vi "PPR_Teleop_System_Execute.vi"(11 "Teleop Elapsed Seconds":dbl) -> ()   [LabVIEW 2019]
uses:
  <vilib>/Rock Robotics/WPI/Joystick/XBox Buttons Indexer.ctl
  <vilib>/Rock Robotics/WPI/Joystick/XBox Axes Indexer.ctl
  <vilib>/Rock Robotics/WPI/ThirdParty/JAS_Junk/TrajLib/Rotation2d_CreateAngle.vi
  <vilib>/Rock Robotics/WPI/ThirdParty/JAS_Junk/TrajLib/Translation2d_Create.vi
  <vilib>/Rock Robotics/WPI/ThirdParty/JAS_Junk/TrajLib/VI/Util_GetTime_U32.vi
  <vilib>/Rock Robotics/WPI/ThirdParty/JAS_Junk/TrajLib/VI/BoolCmd_Send_Internal.vi
  <vilib>/Rock Robotics/WPI/ThirdParty/JAS_Junk/TrajLib/VI/numCmd_ObtainQueue_TwoDbl.vi
  <vilib>/Rock Robotics/WPI/ThirdParty/JAS_Junk/TrajLib/VI/BoolCmd_ObtainQueue.vi
  <vilib>/Rock Robotics/WPI/ThirdParty/JAS_Junk/TrajLib/VI/Util_GetTime_U64.vi
  Diff_Drive_System/PPR_DRIVE_GLOBALS.vi
  <vilib>/Rock Robotics/WPI/Utilities/WPI_GetSetVariantRefNum.vi
  <vilib>/Rock Robotics/Network Tables/NT Write Integer Array.vi
  Trajectory Following/PPR_TRAJECTORY_GLOBALS.vi
  <vilib>/Rock Robotics/Network Tables/NT Write Numeric Array.vi
  <vilib>/Rock Robotics/WPI/Joystick/WPI_JoystickArcadeMapping.vi
  <vilib>/Rock Robotics/Network Tables/NT Write Boolean Array.vi
  <vilib>/Rock Robotics/WPI/ThirdParty/JAS_Junk/TrajLib/Trajectory_Library.lvlib
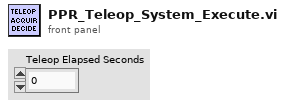
[diagram p1: front panel]
types:
  T1 = typedef "XBox Buttons Indexer.ctl" = enum16{"A", "B", "X", "Y", "Left Bumper", "Right Bumper", "Back", "Start", "Left Joystick", "Right Joystick"}
  T2 = typedef "XBox Axes Indexer.ctl" = enum16{"Left X", "Left Y", "Left Trigger", "Right Trigger", "Right X", "Right Y"}
  T3 = typedef "WPI_JoystickDevRef.ctl" = cluster{"Device":T4}
  T4 = typedef "WPI_JoystickDeviceEnum.ctl" = enum16{"USB 0", "USB 1", "USB 2", "USB 3", "USB 4", "USB 5"}
  T5 = typedef "Trajectory_Library.lvlib/CHASSIS_SPEEDS.ctl" = cluster{"vX":dbl, "vY":dbl, "vOmega":dbl}
  T6 = typedef "Trajectory_Library.lvlib/POSE2D.ctl" = cluster{"TRANSLATION":T7, "ROTATION":T8}
  T7 = typedef "Trajectory_Library.lvlib/TRANSLATION2D.ctl" = cluster{"X":dbl, "Y":dbl}
  T8 = typedef "Trajectory_Library.lvlib/ROTATION2D.ctl" = cluster{"VALUE":dbl, "COS":dbl, "SIN":dbl}
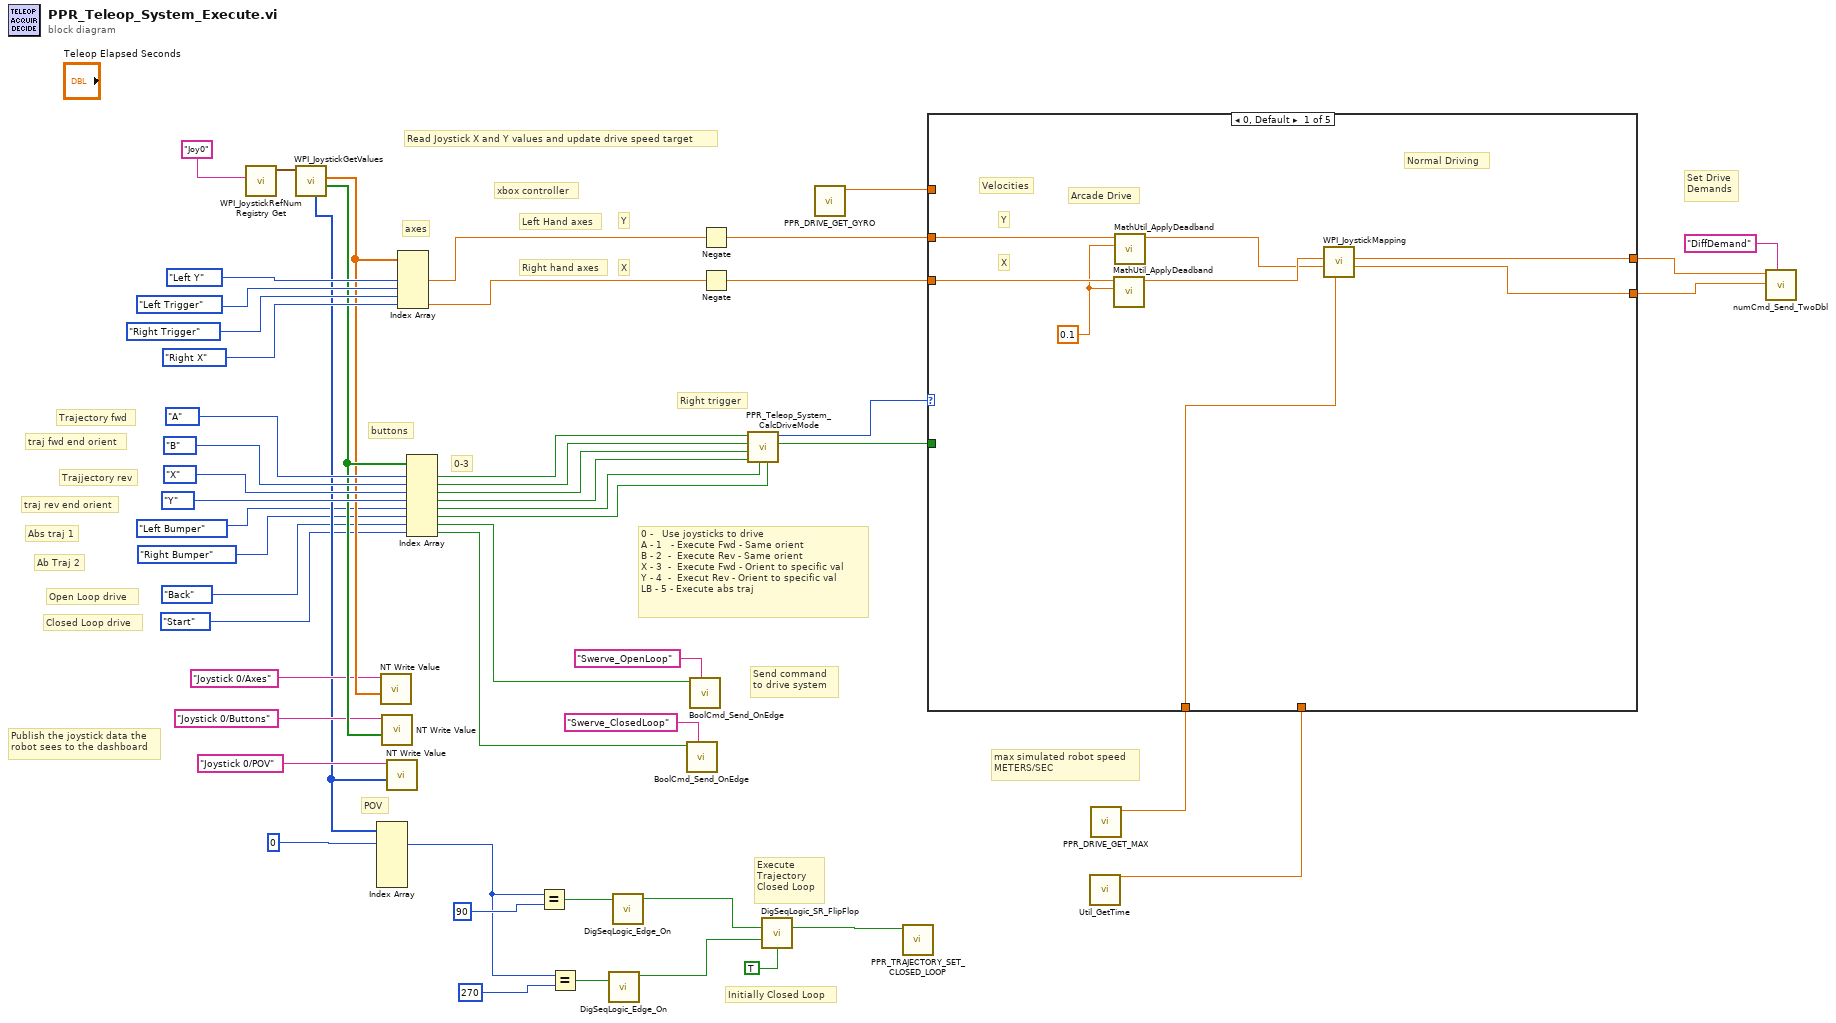
[diagram p0: block diagram]
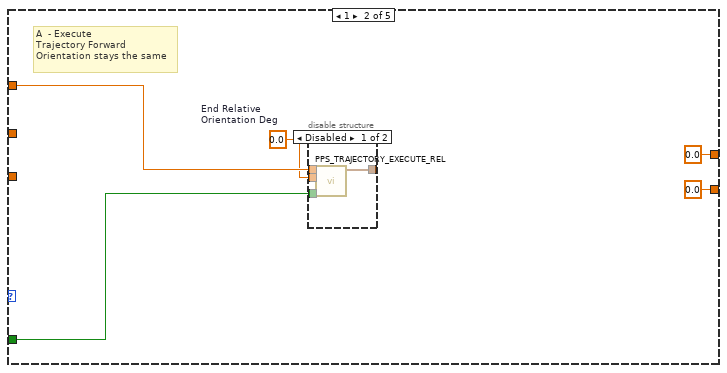
[diagram p2: hidden frame]
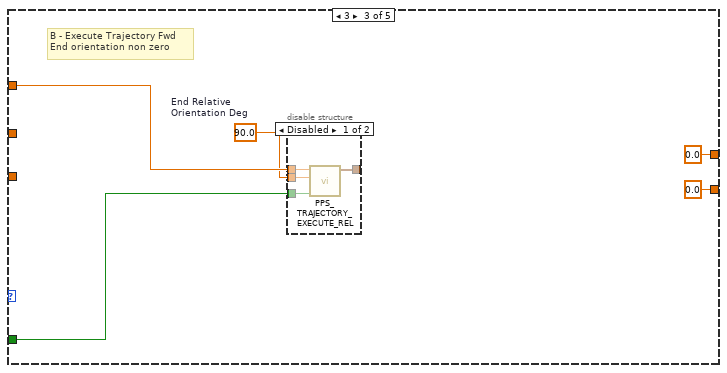
[diagram p4: hidden frame]
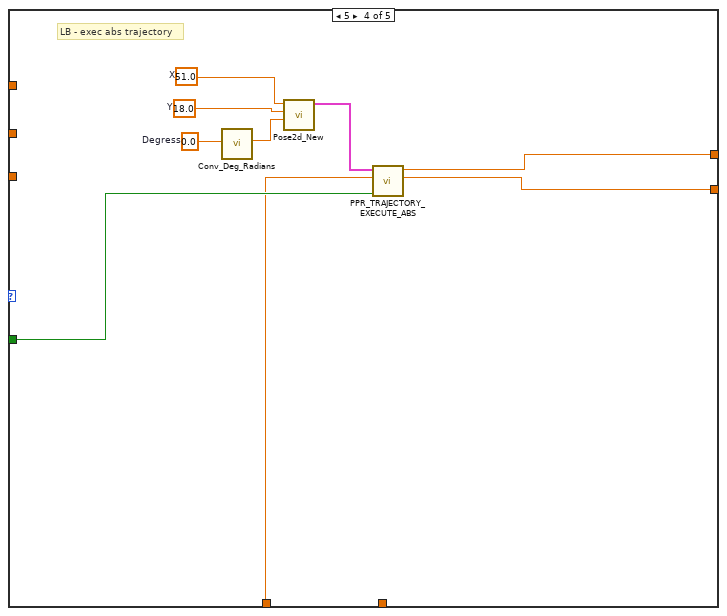
[diagram p6: hidden frame]
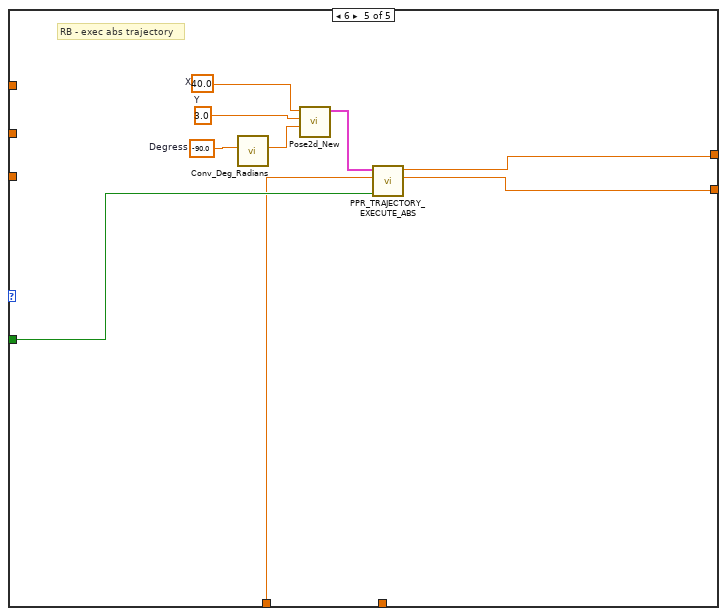
[diagram p7: hidden frame]
diagram:
  # "Send command\nto drive system"
  # "Ab Traj 2"
  # "Abs traj 1"
  # "POV"
  # "traj rev end orient"
  # "traj fwd end orient"
  # "Trajjectory rev"
  # "Closed Loop drive"
  # "Open Loop drive"
  # "Trajectory fwd"
  # "0 -   Use joysticks to drive\nA - 1   - Execute Fwd - Same orient\nB - 2  -  Execute Rev - Same orient\nX - 3  -  Execute Fwd - Orient to specific val\nY - 4  -  Execut Rev - Orient to specific val\nLB - 5 - Execute abs traj"
  # "Execute\nTrajectory\nClosed Loop"
  # "Set Drive\nDemands"
  # "Initially Closed Loop"
  # "0-3"
  # "xbox controller"
  # "Right trigger"
  # "Left Hand axes"
  # "Right hand axes"
  # "X"
  # "Y"
  # "buttons"
  # "axes"
  # "max simulated robot speed\nMETERS/SEC"
  # "Publish the joystick data the\nrobot sees to the dashboard"
  # "Read Joystick X and Y values and update drive speed target"
  n1 = call <vilib>:"WPI_JoystickRefNum Registry Get.vi"("refnum name"="Joy0") -> ("JoystickDevRef"=w27:T3)  [unwired: 1 in, 9 out]
  n2 = call <vilib>:"WPI_JoystickGetValues.vi"("JoystickDevRef"=w27) -> ("Buttons"=w31:bool[], "Axes"=w30:dbl[], "POVs"=w21:i16[])  [unwired: 6 in, 2 out]
  n3 = Index Array(array=w21, index #1=0 ("index")) -> (element #1=w17:i16)  [unwired: 5 in, 5 out]
  n4 = call-poly <vilib>:"NT Write Value.vi"("value"=w30, "name"="Joystick 0/Axes" ("Name")) -> ()  [unwired: 9 in, 1 out]
  n5 = call-poly <vilib>:"NT Write Value.vi"("value"=w31, "name"="Joystick 0/Buttons" ("Name")) -> ()  [unwired: 9 in, 1 out]
  n6 = call-poly <vilib>:"NT Write Value.vi"("value"=w21, "name"="Joystick 0/POV" ("Name")) -> ()  [unwired: 9 in, 1 out]
  n7 = Index Array(array=w30, index #2=XBox_Axes_Indexer."Left Y" ("XBox Axes"), index #3=XBox_Axes_Indexer."Left Trigger" ("XBox Axes"), index #4=XBox_Axes_Indexer."Right Trigger" ("XBox Axes"), index #5=XBox_Axes_Indexer."Right X" ("XBox Axes")) -> (element #2=w38:dbl, element #5=w39:dbl)  [unwired: 1 in, 3 out]
  n8 = Index Array(array=w31, index #1=XBox_Buttons_Indexer."A" ("XBox Buttons"), index #2=XBox_Buttons_Indexer."B" ("XBox Buttons"), index #3=XBox_Buttons_Indexer."X" ("XBox Buttons"), index #4=XBox_Buttons_Indexer."Y" ("XBox Buttons"), index #5=XBox_Buttons_Indexer."Left Bumper" ("XBox Buttons"), index #6=XBox_Buttons_Indexer."Right Bumper" ("XBox Buttons"), index #7=XBox_Buttons_Indexer."Back" ("XBox Buttons"), index #8=XBox_Buttons_Indexer."Start" ("XBox Buttons")) -> (element #1=w32:bool, element #2=w40:bool, element #3=w41:bool, element #4=w48:bool, element #5=w8:bool, element #6=w7:bool, element #7=w4:bool, element #8=w3:bool)
  n9 = Equal?(x=w17, y=i16 90) -> (x = y?=w16:bool)
  n10 = Equal?(x=w17, y=i16 270) -> (x = y?=w15:bool)
  n11 = call <vilib>:"DigSeqLogic_Edge_On.vi"("Input"=w15) -> ("On Edge"=w13:bool)  [unwired: 10 in]
  n12 = call <vilib>:"DigSeqLogic_Edge_On.vi"("Input"=w16) -> ("On Edge"=w14:bool)  [unwired: 10 in]
  n13 = call <vilib>:"BoolCmd_Send_OnEdge.vi"("Command Name"="Swerve_ClosedLoop", "Value"=w3) -> ()  [unwired: 9 in, 1 out]
  n14 = call <vilib>:"BoolCmd_Send_OnEdge.vi"("Command Name"="Swerve_OpenLoop", "Value"=w4) -> ()  [unwired: 9 in, 1 out]
  n15 = Negate(x=w38) -> (-x=w36:dbl)
  n16 = Negate(x=w39) -> (-x=w37:dbl)
  n17 = call "PPR_Teleop_System_CalcDriveMode.vi"("Abs Traj 2"=w7, "Abs Traj 1"=w8, "Traj Rev Follow Orient"=w48, "Traj Rev Same Orient"=w41, "Traj Fwd Follow Orient"=w40, "Traj Fwd Same Orient"=w32) -> ("Dirve Mode Changed"=w34:bool, "Drive Mode"=w33:i32)  [unwired: 4 in]
  n18 = call <vilib>:"DigSeqLogic_SR_FlipFlop.vi"("Set"=w14, "Reset"=w13, "Initial Value"=TRUE) -> ("Output"=w43:bool)  [unwired: 11 in, 1 out]
  n19 = call "PPR_DRIVE_GET_GYRO.vi"() -> ("Gyro Heading Radians"=w24:dbl)  [unwired: 11 in]
  n20 = call "PPR_TRAJECTORY_SET_CLOSED_LOOP.vi"("AUTO_CLOSED_LOOP"=w43) -> ()  [unwired: 11 in]
  n21 = call <vilib>:"Util_GetTime.vi"() -> ("FPGA_Time_Seconds"=w25:dbl)  [unwired: 9 in, 2 out]
  n22 = call "PPR_DRIVE_GET_MAX.vi"() -> ("Max Wheel Vel (Meter/Sec)"=w35:dbl)  [unwired: 10 in, 1 out]
  n23 = case shown="0, Default" w33 {
    tunnel: w37 -> [w59 _ _ _ _]
    tunnel: w35 -> [w57 _ _ w79 w90]
    tunnel: w34 -> [_ w65 w74 w87 w96]
    tunnel: w36 -> [w60 _ _ _ _]
    tunnel: w24 -> [_ w64 w73 _ _]
    tunnel: w25 -> [_ _ _ _ _]
    tunnel: [w56 0.0 ("Left Motor Value") 0.0 ("Left Motor Value") w81 w89] -> w2
    tunnel: [w55 0.0 ("Right Motor Value") 0.0 ("Right Motor Value") w80 w88] -> w1
    frame 0, Default {
      w58 = 0.1 ("Deadband")
      # "Normal Driving"
      # "Velocities"
      # "X"
      # "Y"
      # "Arcade Drive"
      n24 = call <vilib>:"MathUtil_ApplyDeadband.vi"("Deadband"=w58, "Value"=w59) -> ("Result"=w54:dbl)  [unwired: 9 in]
      n25 = call <vilib>:"MathUtil_ApplyDeadband.vi"("Deadband"=w58, "Value"=w60) -> ("Result"=w53:dbl)  [unwired: 9 in]
      n26 = call-poly <vilib>:"WPI_JoystickMapping.vi"("Max Output"=w57, "Y axis value"=w53, "X axis value"=w54) -> ("Right Motor Value"=w55:dbl, "Left Motor Value"=w56:dbl)  [unwired: 7 in]
    }
    frame 1 {
      w63 = 0.0  # End Relative Orientation Deg
      # "A  - Execute\nTrajectory Forward\nOrientation stays the same"
      n27 = disable-structure shown="Disabled" {
        disable-tunnel: w65 -> [w69 _]
        disable-tunnel: [w68 _] -> _
        disable-tunnel: w64 -> [w67 _]
        disable-tunnel: w63 -> [w66 _]
        frame Disabled {
          n28 = call "PPS_TRAJECTORY_EXECUTE_REL.vi"("Init"=w69, "End Relative\nOrientation Deg"=w66, "Gyro Heading\nRAD"=w67) -> ("Chassis Velocity Target SI"=w68:T5)  [unwired: 7 in, 1 out]
        }
        frame Enabled {
        }
      }
    }
    frame 3 {
      w72 = 90.0  # End Relative Orientation Deg
      # "B - Execute Trajectory Fwd \nEnd orientation non zero"
      n29 = disable-structure shown="Disabled" {
        disable-tunnel: w74 -> [w78 _]
        disable-tunnel: [w77 _] -> _
        disable-tunnel: w73 -> [w76 _]
        disable-tunnel: w72 -> [w75 _]
        frame Disabled {
          n30 = call "PPS_TRAJECTORY_EXECUTE_REL.vi"("Init"=w78, "End Relative\nOrientation Deg"=w75, "Gyro Heading\nRAD"=w76) -> ("Chassis Velocity Target SI"=w77:T5)  [unwired: 7 in, 1 out]
        }
        frame Enabled {
        }
      }
    }
    frame 5 {
      w83 = 51.0  # X
      w84 = 18.0  # Y
      w85 = 0.0  # Degress
      # "LB - exec abs trajectory"
      n31 = call <vilib>:"Conv_Deg_Radians.vi"("Degress"=w85) -> ("Radians"=w86:dbl)  [unwired: 10 in]
      n32 = call <vilib>:"Pose2d_New.vi"("Heading"=w86, "Y"=w84, "X"=w83) -> ("out POSe"=w82:T6)  [unwired: 8 in]
      n33 = call "PPR_TRAJECTORY_EXECUTE_ABS.vi"("Init"=w87, "Max Wheel Speed M/S"=w79, "End Pose ENG"=w82) -> ("Right Speed Dmd M/S"=w80:dbl, "Left Speed Dmd M/S"=w81:dbl)  [unwired: 6 in, 1 out]
    }
    frame 6 {
      w92 = 40.0  # X
      w93 = 3.0  # Y
      w94 = -90.0  # Degress
      # "RB - exec abs trajectory"
      n34 = call <vilib>:"Conv_Deg_Radians.vi"("Degress"=w94) -> ("Radians"=w95:dbl)  [unwired: 10 in]
      n35 = call <vilib>:"Pose2d_New.vi"("Heading"=w95, "Y"=w93, "X"=w92) -> ("out POSe"=w91:T6)  [unwired: 8 in]
      n36 = call "PPR_TRAJECTORY_EXECUTE_ABS.vi"("Init"=w96, "Max Wheel Speed M/S"=w90, "End Pose ENG"=w91) -> ("Right Speed Dmd M/S"=w88:dbl, "Left Speed Dmd M/S"=w89:dbl)  [unwired: 6 in, 1 out]
    }
  }
  n37 = call <vilib>:"numCmd_Send_TwoDbl.vi"("Command Name"="DiffDemand", "Value 2"=w1, "Value 1"=w2) -> ()  [unwired: 8 in, 1 out]
